vi "FPGAAddon.SpecialityInputs.Generate.vi"(8 "error in (no error)":errorcluster, 11 "Parameters":T1) -> (0 "error out":errorcluster)   [LabVIEW 2015, in "FPGA Addon Input.lvclass"]
uses:
  FPGA Addon Input.lvclass
  FPGAAddon.SpecialityInputs.Generate.Parameters.ctl
  <vilib>/_script/New VI Object TypeDefs/NewVIObject_LVRelativePositionTypeDef.ctl
  <vilib>/_script/New VI Object TypeDefs/NewVIObject_LVRelativeDirectionTypeDef.ctl
  <vilib>/Utility/miscctls.llb/LVPoint32TypeDef.ctl
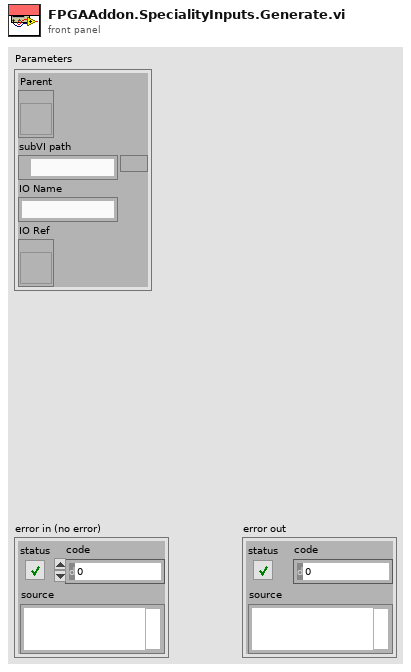
[diagram p1: front panel]
types:
  T1 = typedef "FPGA Addon Input.lvclass/FPGAAddon.SpecialityInputs.Generate.Parameters.ctl" = cluster{"Parent":refnum<vi>, "subVI path":path, "IO Name":string, "IO Ref":refnum<vi>}
  T2 = typedef "NewVIObject_LVRelativePositionTypeDef.ctl" = cluster{"Refnum":refnum<vi>, "Relative Direction":T3, "Point32":T4}
  T3 = typedef "NewVIObject_LVRelativeDirectionTypeDef.ctl" = enum32{"Right", "Left", "Top", "Bottom", "Top Right", "Top Left", "Bottom Right", "Bottom Left"}
  T4 = typedef "LVPoint32TypeDef.ctl" = cluster{"Horizontal":i32, "Vertical":i32}
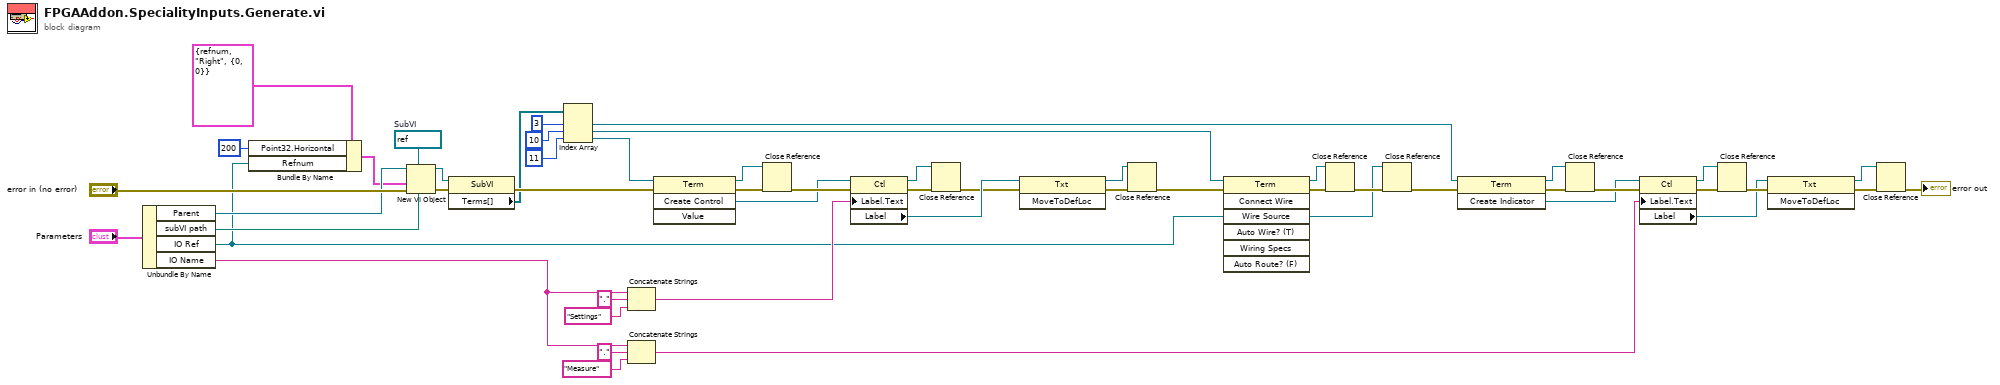
[diagram p0: block diagram]
diagram:
  w22 = refnum<vi> refnum  # SubVI
  n1 = Unbundle By Name("Parameters") -> ("Parent"=w20:refnum<vi>, "subVI path"=w19:path, "IO Ref"=w3:refnum<vi>, "IO Name"=w18:string)
  n2 = Bundle By Name(cluster=T2 {"Refnum"=refnum, "Relative Direction"=enum."Right", "Point32"={"Horizontal"=0, "Vertical"=0}} ("Relative Position"), "Point32.Horizontal"=200, "Refnum"=w3) -> (w1:T2)
  n3 = New VI Object(vi object class=w22, owner refnum=w20, position/next to=w1, 6:w19, 8:"error in (no error)") -> (object refnum=w27:refnum<vi>, 0:w28:errorcluster)  [unwired: 3 in]
  n4 = property class="SubVI"(reference=w27, error in=w28) -> (error out=w29:errorcluster, "Terms[]"=w24:refnum<vi>[])  [unwired: 1 out]
  n5 = Index Array(array=w24, index #1=3 ("index"), index #2=10 ("index"), index #3=11 ("index")) -> (element #1=w42:refnum<vi>, element #2=w33:refnum<vi>, element #3=w43:refnum<vi>)
  n6 = Concatenate Strings(w18, "." ("string"), "Settings" ("string")) -> (w30:string)
  n7 = Concatenate Strings(w18, "." ("string"), "Measure" ("string")) -> (w38:string)
  n8 = invoke class="Term" method="Create Control"(reference=w43, error in=w29) -> (reference out=w40:refnum<vi>, error out=w39:errorcluster, "Create Control"=w17:refnum<vi>)  [unwired: 2 in, 1 out]
  n9 = Close Reference(reference=w40, error in (no error)=w39) -> (error out=w41:errorcluster)
  n10 = property class="Ctl"(reference=w17, error in=w41, "Label.Text"=w30) -> (reference out=w16:refnum<vi>, error out=w14:errorcluster, "Label"=w15:refnum<vi>)
  n11 = Close Reference(reference=w16, error in (no error)=w14) -> (error out=w13:errorcluster)
  n12 = invoke class="Txt" method="MoveToDefLoc"(reference=w15, error in=w13) -> (reference out=w11:refnum<vi>, error out=w12:errorcluster)  [unwired: 1 in, 1 out]
  n13 = Close Reference(reference=w11, error in (no error)=w12) -> (error out=w10:errorcluster)
  n14 = invoke class="Term" method="Connect Wire"(reference=w33, error in=w10, "Wire Source"=w3) -> (reference out=w45:refnum<vi>, error out=w44:errorcluster)  [unwired: 4 in, 5 out]
  n15 = Close Reference(reference=w45, error in (no error)=w44) -> (error out=w46:errorcluster)
  n16 = Close Reference(reference=w3, error in (no error)=w46) -> (error out=w47:errorcluster)
  n17 = invoke class="Term" method="Create Indicator"(reference=w42, error in=w47) -> (reference out=w50:refnum<vi>, error out=w51:errorcluster, "Create Indicator"=w35:refnum<vi>)  [unwired: 1 in]
  n18 = Close Reference(reference=w50, error in (no error)=w51) -> (error out=w52:errorcluster)
  n19 = property class="Ctl"(reference=w35, error in=w52, "Label.Text"=w38) -> (reference out=w48:refnum<vi>, error out=w49:errorcluster, "Label"=w6:refnum<vi>)
  n20 = Close Reference(reference=w48, error in (no error)=w49) -> (error out=w8:errorcluster)
  n21 = invoke class="Txt" method="MoveToDefLoc"(reference=w6, error in=w8) -> (reference out=w5:refnum<vi>, error out=w9:errorcluster)  [unwired: 1 in, 1 out]
  n22 = Close Reference(reference=w5, error in (no error)=w9) -> (error out=→"error out":errorcluster)
